vi "Write Command and Read.vi"(5 "Wait before read (0ms)":u32, 6 "error in (no error)":errorcluster, 7 "Bytes to read (100)":u32=100, 8 "Command":string, 9 "VISA resource name":refnum<visa-resource-name>="COM5") -> (0 "error out":errorcluster, 2 "Returned string":string, 3 "VISA resource name out":refnum<visa-resource-name>="COM5")   [LabVIEW 2020, in "Newport ESP301.lvlib"]
uses:
  Newport ESP301.lvlib
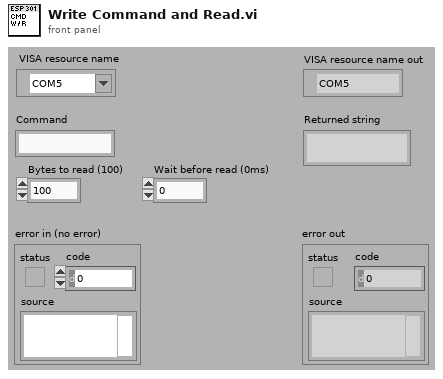
[diagram p1: front panel]
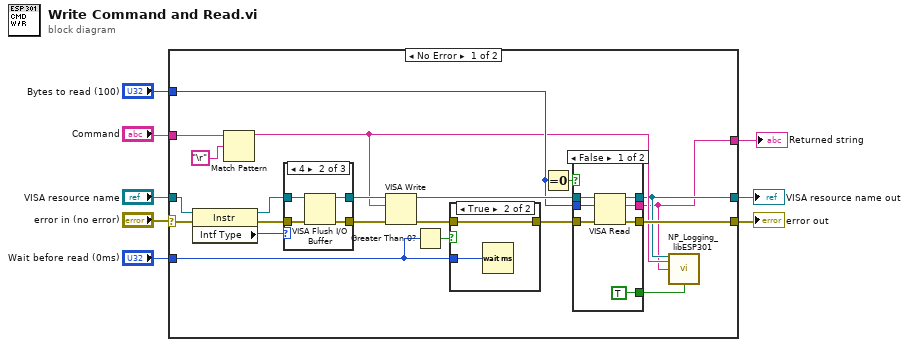
[diagram p0: block diagram]
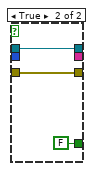
[diagram p4: hidden frame]
diagram:
  n1 = case shown="No Error" "error in (no error)" {
    selector: "error in (no error)" -> [w16 w52]
    tunnel: [w29 w52] -> w7
    tunnel: "VISA resource name" -> [w18 w51]
    tunnel: [w10 w51] -> w5
    tunnel: "Command" -> [w14 _]
    tunnel: "Bytes to read (100)" -> [w21 _]
    tunnel: [w9 _] -> w2
    tunnel: "Wait before read (0ms)" -> [w23 _]
    frame No Error {
      n2 = property class="Instr"(reference=w18, error in=w16) -> (reference out=w17:refnum<visa-resource-name>, error out=w15:errorcluster, "Intf Type"=w19:u16)
      n3 = Match Pattern(string=w14, regular expression="\r") -> (before substring=w11:string)  [unwired: 4 out]
      n4 = case shown="4" w19 {
        tunnel: w17 -> [w31 w33 w37]
        tunnel: [w31 w32 w37] -> w27
        tunnel: w15 -> [w30 w35 w36]
        tunnel: [w30 w34 w36] -> w26
        frame 1 {
        }
        frame 4 {
          n5 = VISA Flush I/O Buffer(VISA resource name=w33, error in (no error)=w35) -> (VISA resource name out=w32:refnum<visa-resource-name>, error out=w34:errorcluster)  [unwired: 1 out]
        }
        frame Default {
        }
      }
      n6 = VISA Write(VISA resource name=w27, write buffer=w11, error in (no error)=w26) -> (VISA resource name out=w28:refnum<visa-resource-name>, error out=w25:errorcluster)  [unwired: 1 out]
      n7 = Greater Than 0?(x=w23) -> (x > 0?=w22:bool)
      n8 = case shown="True" w22 {
        tunnel: w25 -> [w48 w50]
        tunnel: [w48 w50] -> w24
        tunnel: w23 -> [_ w49]
        frame False {
        }
        frame True {
          n9 = Wait (ms)(milliseconds to wait=w49) -> ()  [unwired: 1 out]
        }
      }
      n10 = Equal To 0?(x=w21) -> (x = 0?=w20:bool)
      n11 = case shown="False" w20 {
        tunnel: [w44 w47] -> w29
        tunnel: w28 -> [w43 w46]
        tunnel: [w42 w46] -> w10
        tunnel: w21 -> [w41 _]
        tunnel: [w40 _] -> w9
        tunnel: w24 -> [w39 w47]
        tunnel: [TRUE ("String 2 Enable (T)") FALSE ("String 2 Enable (T)")] -> w12
        frame False {
          n12 = VISA Read(VISA resource name=w43, byte count=w41, error in (no error)=w39) -> (VISA resource name out=w42:refnum<visa-resource-name>, read buffer=w40:string, error out=w44:errorcluster)  [unwired: 1 out]
        }
        frame True {
        }
      }
      n13 = call "NP_Logging_libESP301.vi"("Instrument Channel"=w10, "String 1 {Write} (in)"=w11, "String 2 {Read} (in)"=w9, "String 2 Enable (T)"=w12) -> ()  [unwired: 8 in, 4 out]
    }
    frame Error {
    }
  }
  "error out" <- w7
  "VISA resource name out" <- w5
  "Returned string" <- w2
